vi "7Segment_main_Display.vi"(2 "Time":u32) -> ()   [LabVIEW 2020]
panel:
  out "Boolean 2":bool
  out "Boolean":bool
  out "7Segment1sec":T1
  out "7Segment10sec":T1
  out "7Segment1min":T1
  out "7Segment10min":T1
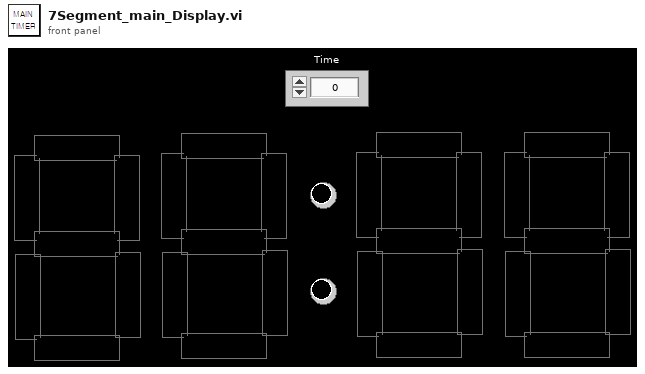
[diagram p1: front panel]
types:
  T1 = cluster{"Led 4":bool, "Led":bool, "Led 3":bool, "Led 2":bool, "Led 5":bool, "Led 6":bool, "Led 7":bool}
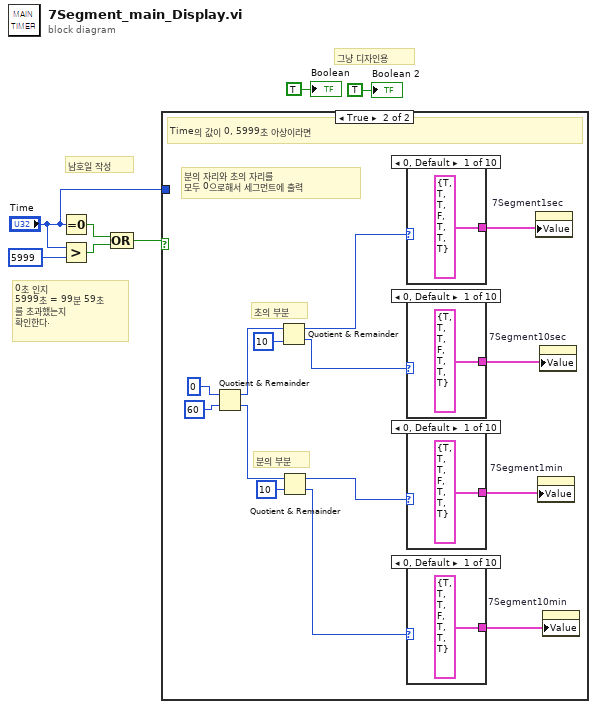
[diagram p0: block diagram]
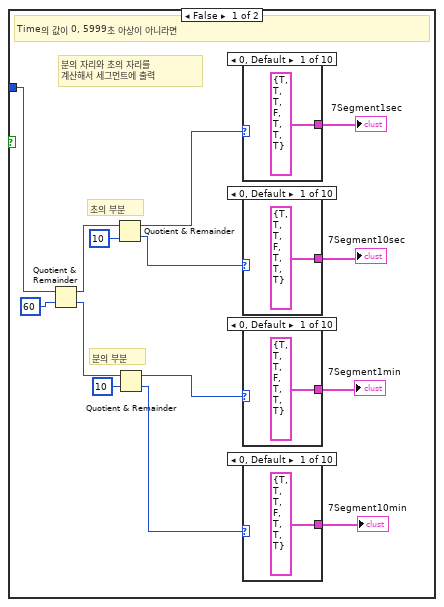
[diagram p2: hidden frame]
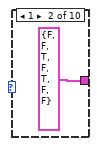
[diagram p3: hidden frame]
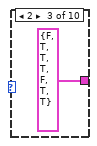
[diagram p4: hidden frame]
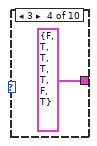
[diagram p5: hidden frame]
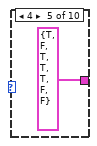
[diagram p6: hidden frame]
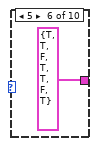
[diagram p7: hidden frame]
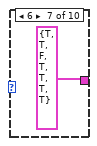
[diagram p8: hidden frame]
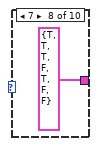
[diagram p9: hidden frame]
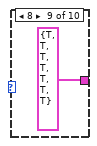
[diagram p10: hidden frame]
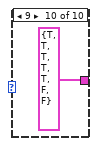
[diagram p11: hidden frame]
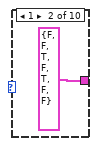
[diagram p12: hidden frame]
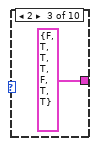
[diagram p13: hidden frame]
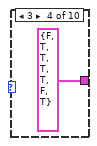
[diagram p14: hidden frame]
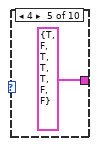
[diagram p15: hidden frame]
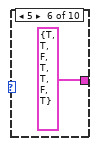
[diagram p16: hidden frame]
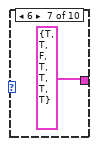
[diagram p17: hidden frame]
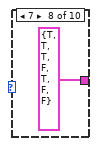
[diagram p18: hidden frame]
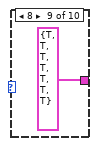
[diagram p19: hidden frame]
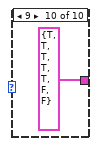
[diagram p20: hidden frame]
diagram:
  # "남호일 작성"
  # "0초 인지\n5999초 = 99분 59초\n를 초과했는지\n확인한다."
  # "그냥 디자인용"
  n1 = Equal To 0?(x="Time") -> (x = 0?=w6:bool)
  n2 = Greater?(x="Time", y=5999) -> (0:w5:bool)
  n3 = Compound Arithmetic op=OR(w6, w5) -> (w4:bool)
  n4 = case shown="True" w4 {
    tunnel: "Time" -> [w21 _]
    frame False {
      # "분의 자리와 초의 자리를 \n계산해서 세그먼트에 출력"
      # "분의 부분"
      # "초의 부분"
      # "Time의 값이 0, 5999초 아상이 아니라면"
      n5 = Quotient & Remainder(x=w21, y=u16 60) -> (x-y*floor(x/y)=w19:u32, floor(x/y)=w17:u32)
      n6 = Quotient & Remainder(x=w19, y=u16 10) -> (x-y*floor(x/y)=w11:u32, floor(x/y)=w12:u32)
      n7 = Quotient & Remainder(x=w17, y=u16 10) -> (x-y*floor(x/y)=w13:u32, floor(x/y)=w15:u32)
      n8 = case shown="0, Default" w11 {
        tunnel: [T1 {"Led 4"=TRUE, "Led"=TRUE, "Led 3"=TRUE, "Led 2"=FALSE, "Led 5"=TRUE, "Led 6"=TRUE, "Led 7"=TRUE} ("7Segment10min") T1 {"Led 4"=FALSE, "Led"=FALSE, "Led 3"=TRUE, "Led 2"=FALSE, "Led 5"=TRUE, "Led 6"=FALSE, "Led 7"=FALSE} ("7Segment10min") T1 {"Led 4"=FALSE, "Led"=TRUE, "Led 3"=TRUE, "Led 2"=TRUE, "Led 5"=FALSE, "Led 6"=TRUE, "Led 7"=TRUE} ("7Segment10min") T1 {"Led 4"=FALSE, "Led"=TRUE, "Led 3"=TRUE, "Led 2"=TRUE, "Led 5"=TRUE, "Led 6"=FALSE, "Led 7"=TRUE} ("7Segment10min") T1 {"Led 4"=TRUE, "Led"=FALSE, "Led 3"=TRUE, "Led 2"=TRUE, "Led 5"=TRUE, "Led 6"=FALSE, "Led 7"=FALSE} ("7Segment10min") T1 {"Led 4"=TRUE, "Led"=TRUE, "Led 3"=FALSE, "Led 2"=TRUE, "Led 5"=TRUE, "Led 6"=FALSE, "Led 7"=TRUE} ("7Segment10min") T1 {"Led 4"=TRUE, "Led"=TRUE, "Led 3"=FALSE, "Led 2"=TRUE, "Led 5"=TRUE, "Led 6"=TRUE, "Led 7"=TRUE} ("7Segment10min") T1 {"Led 4"=TRUE, "Led"=TRUE, "Led 3"=TRUE, "Led 2"=FALSE, "Led 5"=TRUE, "Led 6"=FALSE, "Led 7"=FALSE} ("7Segment10min") T1 {"Led 4"=TRUE, "Led"=TRUE, "Led 3"=TRUE, "Led 2"=TRUE, "Led 5"=TRUE, "Led 6"=TRUE, "Led 7"=TRUE} ("7Segment10min") T1 {"Led 4"=TRUE, "Led"=TRUE, "Led 3"=TRUE, "Led 2"=TRUE, "Led 5"=TRUE, "Led 6"=FALSE, "Led 7"=FALSE} ("7Segment10min")] -> w8
        frame 0, Default {
        }
        frame 1 {
        }
        frame 2 {
        }
        frame 3 {
        }
        frame 4 {
        }
        frame 5 {
        }
        frame 6 {
        }
        frame 7 {
        }
        frame 8 {
        }
        frame 9 {
        }
      }
      "7Segment1sec" <- w8
      n9 = case shown="0, Default" w12 {
        tunnel: [T1 {"Led 4"=TRUE, "Led"=TRUE, "Led 3"=TRUE, "Led 2"=FALSE, "Led 5"=TRUE, "Led 6"=TRUE, "Led 7"=TRUE} ("7Segment10min") T1 {"Led 4"=FALSE, "Led"=FALSE, "Led 3"=TRUE, "Led 2"=FALSE, "Led 5"=TRUE, "Led 6"=FALSE, "Led 7"=FALSE} ("7Segment10min") T1 {"Led 4"=FALSE, "Led"=TRUE, "Led 3"=TRUE, "Led 2"=TRUE, "Led 5"=FALSE, "Led 6"=TRUE, "Led 7"=TRUE} ("7Segment10min") T1 {"Led 4"=FALSE, "Led"=TRUE, "Led 3"=TRUE, "Led 2"=TRUE, "Led 5"=TRUE, "Led 6"=FALSE, "Led 7"=TRUE} ("7Segment10min") T1 {"Led 4"=TRUE, "Led"=FALSE, "Led 3"=TRUE, "Led 2"=TRUE, "Led 5"=TRUE, "Led 6"=FALSE, "Led 7"=FALSE} ("7Segment10min") T1 {"Led 4"=TRUE, "Led"=TRUE, "Led 3"=FALSE, "Led 2"=TRUE, "Led 5"=TRUE, "Led 6"=FALSE, "Led 7"=TRUE} ("7Segment10min") T1 {"Led 4"=TRUE, "Led"=TRUE, "Led 3"=FALSE, "Led 2"=TRUE, "Led 5"=TRUE, "Led 6"=TRUE, "Led 7"=TRUE} ("7Segment10min") T1 {"Led 4"=TRUE, "Led"=TRUE, "Led 3"=TRUE, "Led 2"=FALSE, "Led 5"=TRUE, "Led 6"=FALSE, "Led 7"=FALSE} ("7Segment10min") T1 {"Led 4"=TRUE, "Led"=TRUE, "Led 3"=TRUE, "Led 2"=TRUE, "Led 5"=TRUE, "Led 6"=TRUE, "Led 7"=TRUE} ("7Segment10min") T1 {"Led 4"=TRUE, "Led"=TRUE, "Led 3"=TRUE, "Led 2"=TRUE, "Led 5"=TRUE, "Led 6"=FALSE, "Led 7"=FALSE} ("7Segment10min")] -> w9
        frame 0, Default {
        }
        frame 1 {
        }
        frame 2 {
        }
        frame 3 {
        }
        frame 4 {
        }
        frame 5 {
        }
        frame 6 {
        }
        frame 7 {
        }
        frame 8 {
        }
        frame 9 {
        }
      }
      "7Segment10sec" <- w9
      n10 = case shown="0, Default" w13 {
        tunnel: [T1 {"Led 4"=TRUE, "Led"=TRUE, "Led 3"=TRUE, "Led 2"=FALSE, "Led 5"=TRUE, "Led 6"=TRUE, "Led 7"=TRUE} ("7Segment10min") T1 {"Led 4"=FALSE, "Led"=FALSE, "Led 3"=TRUE, "Led 2"=FALSE, "Led 5"=TRUE, "Led 6"=FALSE, "Led 7"=FALSE} ("7Segment10min") T1 {"Led 4"=FALSE, "Led"=TRUE, "Led 3"=TRUE, "Led 2"=TRUE, "Led 5"=FALSE, "Led 6"=TRUE, "Led 7"=TRUE} ("7Segment10min") T1 {"Led 4"=FALSE, "Led"=TRUE, "Led 3"=TRUE, "Led 2"=TRUE, "Led 5"=TRUE, "Led 6"=FALSE, "Led 7"=TRUE} ("7Segment10min") T1 {"Led 4"=TRUE, "Led"=FALSE, "Led 3"=TRUE, "Led 2"=TRUE, "Led 5"=TRUE, "Led 6"=FALSE, "Led 7"=FALSE} ("7Segment10min") T1 {"Led 4"=TRUE, "Led"=TRUE, "Led 3"=FALSE, "Led 2"=TRUE, "Led 5"=TRUE, "Led 6"=FALSE, "Led 7"=TRUE} ("7Segment10min") T1 {"Led 4"=TRUE, "Led"=TRUE, "Led 3"=FALSE, "Led 2"=TRUE, "Led 5"=TRUE, "Led 6"=TRUE, "Led 7"=TRUE} ("7Segment10min") T1 {"Led 4"=TRUE, "Led"=TRUE, "Led 3"=TRUE, "Led 2"=FALSE, "Led 5"=TRUE, "Led 6"=FALSE, "Led 7"=FALSE} ("7Segment10min") T1 {"Led 4"=TRUE, "Led"=TRUE, "Led 3"=TRUE, "Led 2"=TRUE, "Led 5"=TRUE, "Led 6"=TRUE, "Led 7"=TRUE} ("7Segment10min") T1 {"Led 4"=TRUE, "Led"=TRUE, "Led 3"=TRUE, "Led 2"=TRUE, "Led 5"=TRUE, "Led 6"=FALSE, "Led 7"=FALSE} ("7Segment10min")] -> w10
        frame 0, Default {
        }
        frame 1 {
        }
        frame 2 {
        }
        frame 3 {
        }
        frame 4 {
        }
        frame 5 {
        }
        frame 6 {
        }
        frame 7 {
        }
        frame 8 {
        }
        frame 9 {
        }
      }
      "7Segment1min" <- w10
      n11 = case shown="0, Default" w15 {
        tunnel: [T1 {"Led 4"=TRUE, "Led"=TRUE, "Led 3"=TRUE, "Led 2"=FALSE, "Led 5"=TRUE, "Led 6"=TRUE, "Led 7"=TRUE} ("7Segment10min") T1 {"Led 4"=FALSE, "Led"=FALSE, "Led 3"=TRUE, "Led 2"=FALSE, "Led 5"=TRUE, "Led 6"=FALSE, "Led 7"=FALSE} ("7Segment10min") T1 {"Led 4"=FALSE, "Led"=TRUE, "Led 3"=TRUE, "Led 2"=TRUE, "Led 5"=FALSE, "Led 6"=TRUE, "Led 7"=TRUE} ("7Segment10min") T1 {"Led 4"=FALSE, "Led"=TRUE, "Led 3"=TRUE, "Led 2"=TRUE, "Led 5"=TRUE, "Led 6"=FALSE, "Led 7"=TRUE} ("7Segment10min") T1 {"Led 4"=TRUE, "Led"=FALSE, "Led 3"=TRUE, "Led 2"=TRUE, "Led 5"=TRUE, "Led 6"=FALSE, "Led 7"=FALSE} ("7Segment10min") T1 {"Led 4"=TRUE, "Led"=TRUE, "Led 3"=FALSE, "Led 2"=TRUE, "Led 5"=TRUE, "Led 6"=FALSE, "Led 7"=TRUE} ("7Segment10min") T1 {"Led 4"=TRUE, "Led"=TRUE, "Led 3"=FALSE, "Led 2"=TRUE, "Led 5"=TRUE, "Led 6"=TRUE, "Led 7"=TRUE} ("7Segment10min") T1 {"Led 4"=TRUE, "Led"=TRUE, "Led 3"=TRUE, "Led 2"=FALSE, "Led 5"=TRUE, "Led 6"=FALSE, "Led 7"=FALSE} ("7Segment10min") T1 {"Led 4"=TRUE, "Led"=TRUE, "Led 3"=TRUE, "Led 2"=TRUE, "Led 5"=TRUE, "Led 6"=TRUE, "Led 7"=TRUE} ("7Segment10min") T1 {"Led 4"=TRUE, "Led"=TRUE, "Led 3"=TRUE, "Led 2"=TRUE, "Led 5"=TRUE, "Led 6"=FALSE, "Led 7"=FALSE} ("7Segment10min")] -> w14
        frame 0, Default {
        }
        frame 1 {
        }
        frame 2 {
        }
        frame 3 {
        }
        frame 4 {
        }
        frame 5 {
        }
        frame 6 {
        }
        frame 7 {
        }
        frame 8 {
        }
        frame 9 {
        }
      }
      "7Segment10min" <- w14
    }
    frame True {
      # "분의 자리와 초의 자리를 \n모두 0으로해서 세그먼트에 출력"
      # "분의 부분"
      # "초의 부분"
      # "Time의 값이 0, 5999초 아상이라면"
      n12 = Quotient & Remainder(x=u16 0, y=u16 60) -> (x-y*floor(x/y)=w75:u16, floor(x/y)=w74:u16)
      n13 = Quotient & Remainder(x=w75, y=u16 10) -> (x-y*floor(x/y)=w70:u16, floor(x/y)=w71:u16)
      n14 = Quotient & Remainder(x=w74, y=u16 10) -> (x-y*floor(x/y)=w72:u16, floor(x/y)=w73:u16)
      n15 = case shown="0, Default" w70 {
        tunnel: [T1 {"Led 4"=TRUE, "Led"=TRUE, "Led 3"=TRUE, "Led 2"=FALSE, "Led 5"=TRUE, "Led 6"=TRUE, "Led 7"=TRUE} ("7Segment10min") T1 {"Led 4"=FALSE, "Led"=FALSE, "Led 3"=TRUE, "Led 2"=FALSE, "Led 5"=TRUE, "Led 6"=FALSE, "Led 7"=FALSE} ("7Segment10min") T1 {"Led 4"=FALSE, "Led"=TRUE, "Led 3"=TRUE, "Led 2"=TRUE, "Led 5"=FALSE, "Led 6"=TRUE, "Led 7"=TRUE} ("7Segment10min") T1 {"Led 4"=FALSE, "Led"=TRUE, "Led 3"=TRUE, "Led 2"=TRUE, "Led 5"=TRUE, "Led 6"=FALSE, "Led 7"=TRUE} ("7Segment10min") T1 {"Led 4"=TRUE, "Led"=FALSE, "Led 3"=TRUE, "Led 2"=TRUE, "Led 5"=TRUE, "Led 6"=FALSE, "Led 7"=FALSE} ("7Segment10min") T1 {"Led 4"=TRUE, "Led"=TRUE, "Led 3"=FALSE, "Led 2"=TRUE, "Led 5"=TRUE, "Led 6"=FALSE, "Led 7"=TRUE} ("7Segment10min") T1 {"Led 4"=TRUE, "Led"=TRUE, "Led 3"=FALSE, "Led 2"=TRUE, "Led 5"=TRUE, "Led 6"=TRUE, "Led 7"=TRUE} ("7Segment10min") T1 {"Led 4"=TRUE, "Led"=TRUE, "Led 3"=TRUE, "Led 2"=FALSE, "Led 5"=TRUE, "Led 6"=FALSE, "Led 7"=FALSE} ("7Segment10min") T1 {"Led 4"=TRUE, "Led"=TRUE, "Led 3"=TRUE, "Led 2"=TRUE, "Led 5"=TRUE, "Led 6"=TRUE, "Led 7"=TRUE} ("7Segment10min") T1 {"Led 4"=TRUE, "Led"=TRUE, "Led 3"=TRUE, "Led 2"=TRUE, "Led 5"=TRUE, "Led 6"=FALSE, "Led 7"=FALSE} ("7Segment10min")] -> w65
        frame 0, Default {
        }
        frame 1 {
        }
        frame 2 {
        }
        frame 3 {
        }
        frame 4 {
        }
        frame 5 {
        }
        frame 6 {
        }
        frame 7 {
        }
        frame 8 {
        }
        frame 9 {
        }
      }
      n16 = case shown="0, Default" w71 {
        tunnel: [T1 {"Led 4"=TRUE, "Led"=TRUE, "Led 3"=TRUE, "Led 2"=FALSE, "Led 5"=TRUE, "Led 6"=TRUE, "Led 7"=TRUE} ("7Segment10min") T1 {"Led 4"=FALSE, "Led"=FALSE, "Led 3"=TRUE, "Led 2"=FALSE, "Led 5"=TRUE, "Led 6"=FALSE, "Led 7"=FALSE} ("7Segment10min") T1 {"Led 4"=FALSE, "Led"=TRUE, "Led 3"=TRUE, "Led 2"=TRUE, "Led 5"=FALSE, "Led 6"=TRUE, "Led 7"=TRUE} ("7Segment10min") T1 {"Led 4"=FALSE, "Led"=TRUE, "Led 3"=TRUE, "Led 2"=TRUE, "Led 5"=TRUE, "Led 6"=FALSE, "Led 7"=TRUE} ("7Segment10min") T1 {"Led 4"=TRUE, "Led"=FALSE, "Led 3"=TRUE, "Led 2"=TRUE, "Led 5"=TRUE, "Led 6"=FALSE, "Led 7"=FALSE} ("7Segment10min") T1 {"Led 4"=TRUE, "Led"=TRUE, "Led 3"=FALSE, "Led 2"=TRUE, "Led 5"=TRUE, "Led 6"=FALSE, "Led 7"=TRUE} ("7Segment10min") T1 {"Led 4"=TRUE, "Led"=TRUE, "Led 3"=FALSE, "Led 2"=TRUE, "Led 5"=TRUE, "Led 6"=TRUE, "Led 7"=TRUE} ("7Segment10min") T1 {"Led 4"=TRUE, "Led"=TRUE, "Led 3"=TRUE, "Led 2"=FALSE, "Led 5"=TRUE, "Led 6"=FALSE, "Led 7"=FALSE} ("7Segment10min") T1 {"Led 4"=TRUE, "Led"=TRUE, "Led 3"=TRUE, "Led 2"=TRUE, "Led 5"=TRUE, "Led 6"=TRUE, "Led 7"=TRUE} ("7Segment10min") T1 {"Led 4"=TRUE, "Led"=TRUE, "Led 3"=TRUE, "Led 2"=TRUE, "Led 5"=TRUE, "Led 6"=FALSE, "Led 7"=FALSE} ("7Segment10min")] -> w64
        frame 0, Default {
        }
        frame 1 {
        }
        frame 2 {
        }
        frame 3 {
        }
        frame 4 {
        }
        frame 5 {
        }
        frame 6 {
        }
        frame 7 {
        }
        frame 8 {
        }
        frame 9 {
        }
      }
      n17 = case shown="0, Default" w72 {
        tunnel: [T1 {"Led 4"=TRUE, "Led"=TRUE, "Led 3"=TRUE, "Led 2"=FALSE, "Led 5"=TRUE, "Led 6"=TRUE, "Led 7"=TRUE} ("7Segment10min") T1 {"Led 4"=FALSE, "Led"=FALSE, "Led 3"=TRUE, "Led 2"=FALSE, "Led 5"=TRUE, "Led 6"=FALSE, "Led 7"=FALSE} ("7Segment10min") T1 {"Led 4"=FALSE, "Led"=TRUE, "Led 3"=TRUE, "Led 2"=TRUE, "Led 5"=FALSE, "Led 6"=TRUE, "Led 7"=TRUE} ("7Segment10min") T1 {"Led 4"=FALSE, "Led"=TRUE, "Led 3"=TRUE, "Led 2"=TRUE, "Led 5"=TRUE, "Led 6"=FALSE, "Led 7"=TRUE} ("7Segment10min") T1 {"Led 4"=TRUE, "Led"=FALSE, "Led 3"=TRUE, "Led 2"=TRUE, "Led 5"=TRUE, "Led 6"=FALSE, "Led 7"=FALSE} ("7Segment10min") T1 {"Led 4"=TRUE, "Led"=TRUE, "Led 3"=FALSE, "Led 2"=TRUE, "Led 5"=TRUE, "Led 6"=FALSE, "Led 7"=TRUE} ("7Segment10min") T1 {"Led 4"=TRUE, "Led"=TRUE, "Led 3"=FALSE, "Led 2"=TRUE, "Led 5"=TRUE, "Led 6"=TRUE, "Led 7"=TRUE} ("7Segment10min") T1 {"Led 4"=TRUE, "Led"=TRUE, "Led 3"=TRUE, "Led 2"=FALSE, "Led 5"=TRUE, "Led 6"=FALSE, "Led 7"=FALSE} ("7Segment10min") T1 {"Led 4"=TRUE, "Led"=TRUE, "Led 3"=TRUE, "Led 2"=TRUE, "Led 5"=TRUE, "Led 6"=TRUE, "Led 7"=TRUE} ("7Segment10min") T1 {"Led 4"=TRUE, "Led"=TRUE, "Led 3"=TRUE, "Led 2"=TRUE, "Led 5"=TRUE, "Led 6"=FALSE, "Led 7"=FALSE} ("7Segment10min")] -> w63
        frame 0, Default {
        }
        frame 1 {
        }
        frame 2 {
        }
        frame 3 {
        }
        frame 4 {
        }
        frame 5 {
        }
        frame 6 {
        }
        frame 7 {
        }
        frame 8 {
        }
        frame 9 {
        }
      }
      n18 = case shown="0, Default" w73 {
        tunnel: [T1 {"Led 4"=TRUE, "Led"=TRUE, "Led 3"=TRUE, "Led 2"=FALSE, "Led 5"=TRUE, "Led 6"=TRUE, "Led 7"=TRUE} ("7Segment10min") T1 {"Led 4"=FALSE, "Led"=FALSE, "Led 3"=TRUE, "Led 2"=FALSE, "Led 5"=TRUE, "Led 6"=FALSE, "Led 7"=FALSE} ("7Segment10min") T1 {"Led 4"=FALSE, "Led"=TRUE, "Led 3"=TRUE, "Led 2"=TRUE, "Led 5"=FALSE, "Led 6"=TRUE, "Led 7"=TRUE} ("7Segment10min") T1 {"Led 4"=FALSE, "Led"=TRUE, "Led 3"=TRUE, "Led 2"=TRUE, "Led 5"=TRUE, "Led 6"=FALSE, "Led 7"=TRUE} ("7Segment10min") T1 {"Led 4"=TRUE, "Led"=FALSE, "Led 3"=TRUE, "Led 2"=TRUE, "Led 5"=TRUE, "Led 6"=FALSE, "Led 7"=FALSE} ("7Segment10min") T1 {"Led 4"=TRUE, "Led"=TRUE, "Led 3"=FALSE, "Led 2"=TRUE, "Led 5"=TRUE, "Led 6"=FALSE, "Led 7"=TRUE} ("7Segment10min") T1 {"Led 4"=TRUE, "Led"=TRUE, "Led 3"=FALSE, "Led 2"=TRUE, "Led 5"=TRUE, "Led 6"=TRUE, "Led 7"=TRUE} ("7Segment10min") T1 {"Led 4"=TRUE, "Led"=TRUE, "Led 3"=TRUE, "Led 2"=FALSE, "Led 5"=TRUE, "Led 6"=FALSE, "Led 7"=FALSE} ("7Segment10min") T1 {"Led 4"=TRUE, "Led"=TRUE, "Led 3"=TRUE, "Led 2"=TRUE, "Led 5"=TRUE, "Led 6"=TRUE, "Led 7"=TRUE} ("7Segment10min") T1 {"Led 4"=TRUE, "Led"=TRUE, "Led 3"=TRUE, "Led 2"=TRUE, "Led 5"=TRUE, "Led 6"=FALSE, "Led 7"=FALSE} ("7Segment10min")] -> w62
        frame 0, Default {
        }
        frame 1 {
        }
        frame 2 {
        }
        frame 3 {
        }
        frame 4 {
        }
        frame 5 {
        }
        frame 6 {
        }
        frame 7 {
        }
        frame 8 {
        }
        frame 9 {
        }
      }
      n19 = property on="7Segment1sec" class="Clust (strict)"("Value"=w65) -> ()  [unwired: 2 in, 2 out]
      n20 = property on="7Segment1min" class="Clust (strict)"("Value"=w63) -> ()  [unwired: 2 in, 2 out]
      n21 = property on="7Segment10sec" class="Clust (strict)"("Value"=w64) -> ()  [unwired: 2 in, 2 out]
      n22 = property on="7Segment10min" class="Clust (strict)"("Value"=w62) -> ()  [unwired: 2 in, 2 out]
    }
  }
  "Boolean" <- TRUE ("Boolean")
  "Boolean 2" <- TRUE ("Boolean 2")
